vi "Demodulator.vi"(5 "Initial df":dbl, 7 "rx":cdb[](array[numeric]), 9 "I*":cdb[](array[numeric])) -> (8 "all symbols":cdb[][](array[numeric]))   [LabVIEW 2017]
uses:
  <vilib>/Analysis/2dsp.llb/Upsample (CDB).vi
  <vilib>/Analysis/3filter.llb/FIR Filter (CDB).vi
  <vilib>/Analysis/NI_AALBase.lvlib
  <vilib>/Analysis/NI_AALPro.lvlib
panel:
  out "df corr":dbl format="%0.2f"
  out "b":dbl format="%0.2f"
  out "a":dbl
  in  "discr":cdb[](array[numeric])
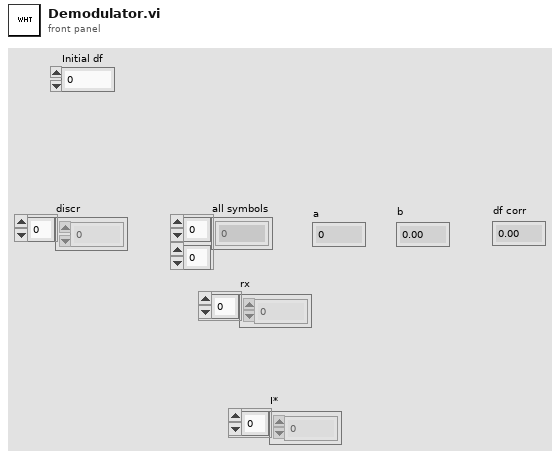
[diagram p1: front panel]
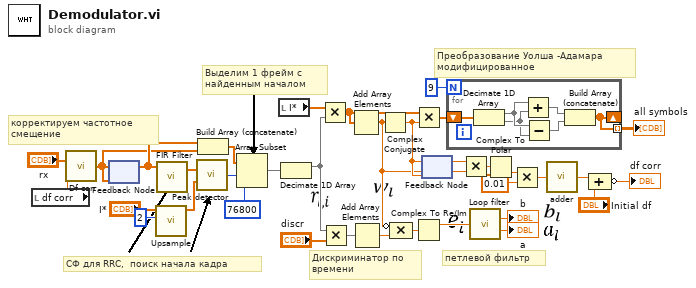
[diagram p0: block diagram]
diagram:
  # "петлевой фильтр"
  # "корректируем частотное \nсмещение"
  # "Выделим 1 фрейм с\nнайденным началом"
  # "СФ для RRC,  поиск начала кадра"
  # "Дискриминатор по\nвремени"
  # "Преобразование Уолша -Адамара\nмодифицированное"
  n1 = local read "df corr"() -> (w5:dbl)
  n2 = call "Df corr.vi"("in"="rx", "df"=w5) -> ("out"=w6:cdb[])  [unwired: 13 in]
  n3 = feedback #1(w6) -> (w15:cdb[])
  n4 = feedback-in #1(w6) -> ()
  n5 = call-poly <vilib>:"Upsample.vi"("upsampling factor"=2, "X"="I*") -> ("Upsampled Array"=w12:cdb[])  [unwired: 8 in, 1 out]
  n6 = call-poly <vilib>:"FIR Filter.vi"("X"=w15) -> ("Filtered X"=w18:cdb[])  [unwired: 3 in, 1 out]
  n7 = call "Peak detector.vi"("X"=w18, "Y"=w12) -> ("peak index"=w9:i32)  [unwired: 11 in, 2 out]
  n8 = Build Array (concatenate)(w15, w6) -> (w17:cdb[])
  n9 = Array Subset(array=w17, index=w9, length=76800) -> (w16:cdb[])
  n10 = local read "I*"() -> (w8:cdb[])
  n11 = Decimate 1D Array(w16) -> (w10:cdb[])  [unwired: 1 out]
  n12 = Multiply(x=w8, y=w10) -> (x*y=w34:cdb[])
  n13 = Multiply(x=w10, y="discr") -> (x*y=w29:cdb[])
  n14 = Add Array Elements(numeric array=w34) -> (sum=w26:cdb)
  n15 = Add Array Elements(numeric array=w29) -> (sum=w27:cdb)
  n16 = Complex Conjugate(1:w26) -> (0:w32:cdb)
  n17 = Compound Arithmetic op=MULTIPLY(invert w26, w27) -> (w24:cdb)
  n18 = Multiply(x=w34, y=w32) -> (x*y=w33:cdb[])
  n19 = Complex To Re/Im(x + iy=w24) -> (x=w20:dbl)  [unwired: 1 out]
  n20 = feedback-in #2(w32) -> ()
  n21 = feedback #2(w32) -> (w31:cdb)
  n22 = for {
    N: 9 -> [_]
    shift-right: [w36] -> _
    shift-left: w33 -> [w41]
    tunnel: [w36] -> w25 mode=indexing
    n23 = Decimate 1D Array(w41) -> (w40:cdb[], w39:cdb[])
    n24 = Add(x=w40, y=w39) -> (x+y=w37:cdb[])
    n25 = Subtract(x=w40, y=w39) -> (x-y=w38:cdb[])
    n26 = Build Array (concatenate)(w37, w38) -> (w36:cdb[])
  }
  "all symbols" <- w25
  n27 = Multiply(x=w31, y=w26) -> (x*y=w30:cdb)
  n28 = call "Loop filter.vi"("e"=w20) -> ("a"=→"b":dbl, "b"=→"a":dbl)  [unwired: 13 in]
  n29 = Complex To Polar(r * e^(i*theta)=w30) -> (theta=w23:dbl)  [unwired: 1 out]
  n30 = Multiply(x=w23, y=0.01) -> (x*y=w21:dbl)
  n31 = call "adder.vi"("x"=w21) -> ("sum"=w3:dbl)  [unwired: 14 in]
  n32 = Compound Arithmetic op=ADD(w3, "Initial df") -> (invert →"df corr":dbl)
